vi "Description.vi"(8 "error in (no error)":errorcluster, 11 "Ignore Inputs Comparator in":refnum<class "Any Inputs Comparator.lvclass">) -> (0 "error out":errorcluster, 2 "Description":string)   [LabVIEW 2020, in "Any Inputs Comparator.lvclass"]
uses:
  Any Inputs Comparator.lvclass
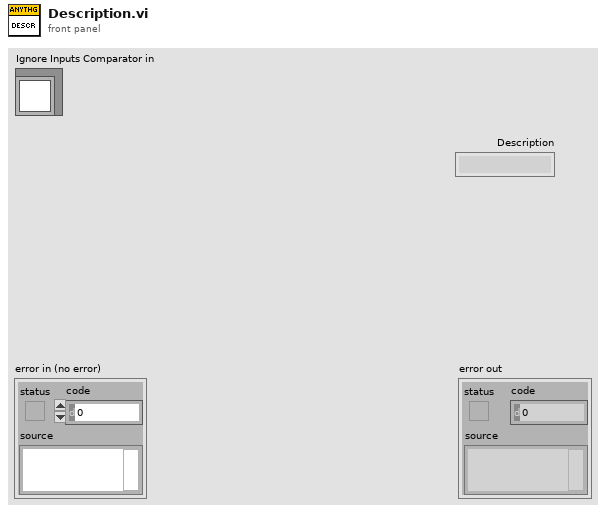
[diagram p1: front panel]
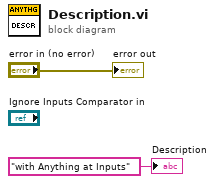
[diagram p0: block diagram]
diagram:
  "error out" <- "error in (no error)"
  "Description" <- "with Anything at Inputs" ("Description")
